vi "Set_valves2.vi"() -> ()   [LabVIEW 2016]
uses:
  ValveGlobals.vi
panel:
  in  "Stop Signal":bool
  out "stop indicator":bool
  in  "Switch Valves":enum16{"1", "2", "3", "4", "5", "6", "7", "8"}[](array[ring])=[enum."6", enum."7"]
  in  "Switch Toggle":bool
  out "Channels 2":bool[][](array[boolean])
  in  "Set Shortcut Pattern":bool
  in  "Clean Cycle Wait Time (s)":u32=8
  in  "Clean Cycle":bool
  in  "Close all Valves":bool
  in  "Set new Values":bool
  in  "stop":bool
  in  "Update Immediately":bool=TRUE
  in  "Which box":string[](array[string])=["A", "B", "C"]
  in  "Channel Nums":string[](array[string])=["1", "2", "3", "4", "5", "6", "7", "8"]
  in  "Channels":bool[][](array[boolean])=[[FALSE, FALSE, FALSE], [FALSE, FALSE, FALSE], [FALSE, FALSE, FALSE], [FALSE, FALSE, FALSE], [FALSE, FALSE, FALSE], [FALSE, FALSE, FALSE], [FALSE, FALSE, FALSE], [FALSE, FALSE, FALSE]]
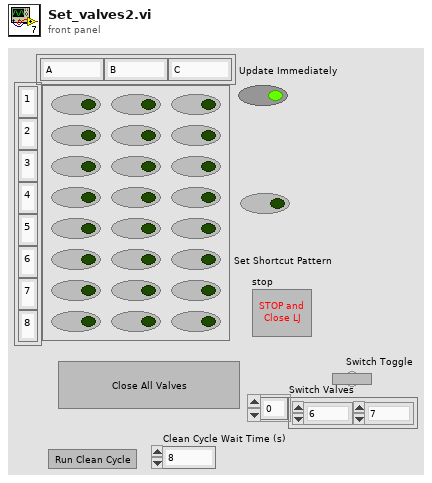
[diagram p1: front panel]
types:
  T1 = enum16{"Release", "Create", "Send", "Wait", "Cancel"}
  T2 = cluster{"Flowboards":enum16{"A", "B", "C"}[], "Channels":enum16{"1", "2", "3", "4", "5", "6", "7", "8"}[], "States":bool[]}
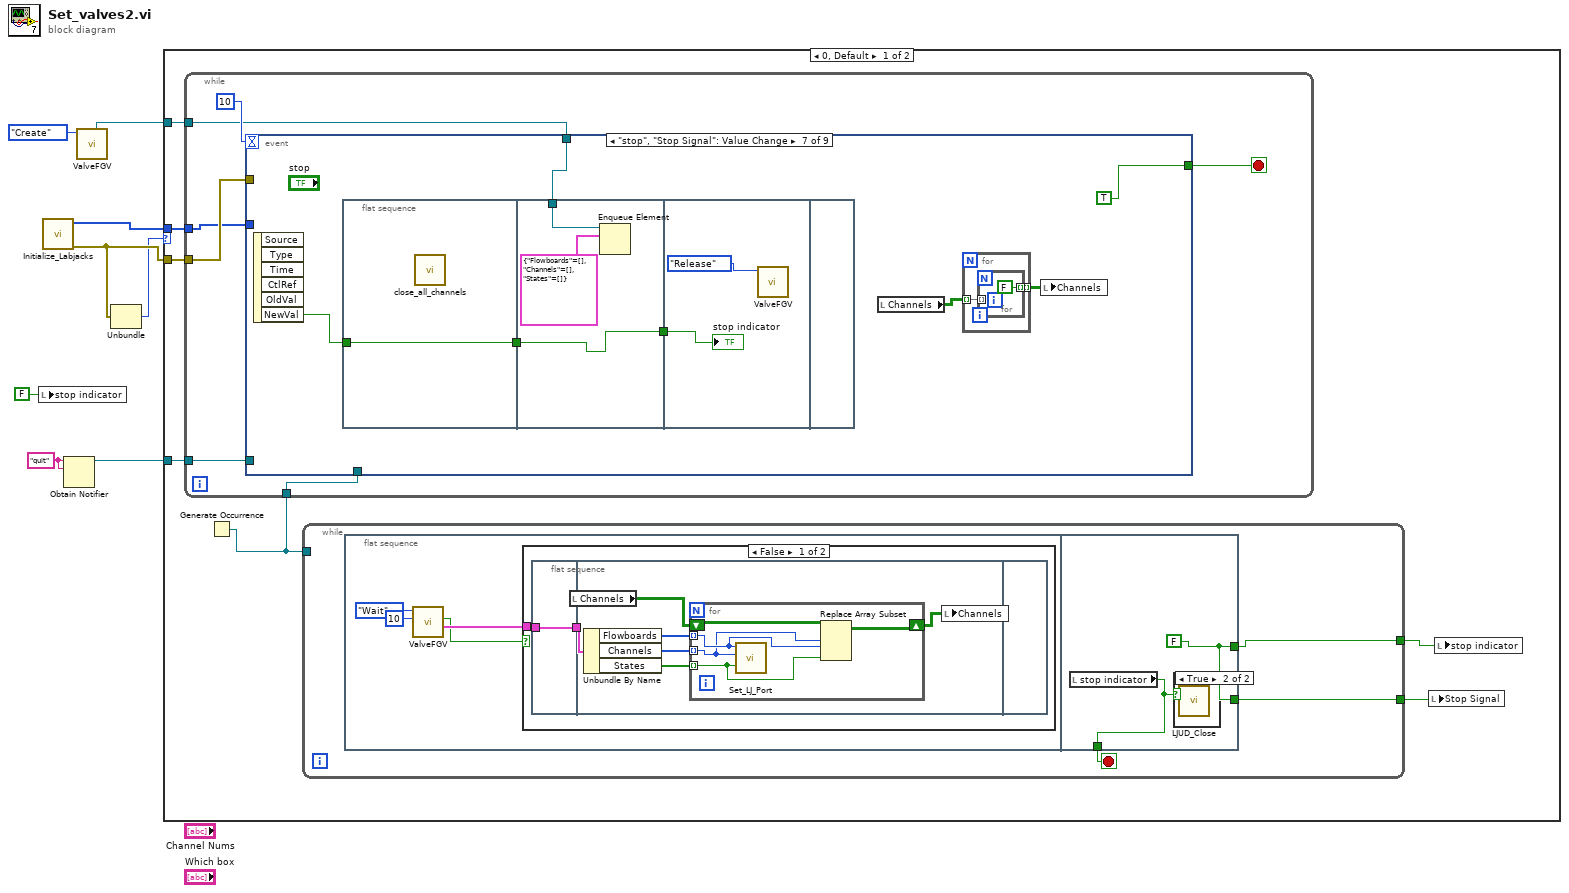
[diagram p0: block diagram]
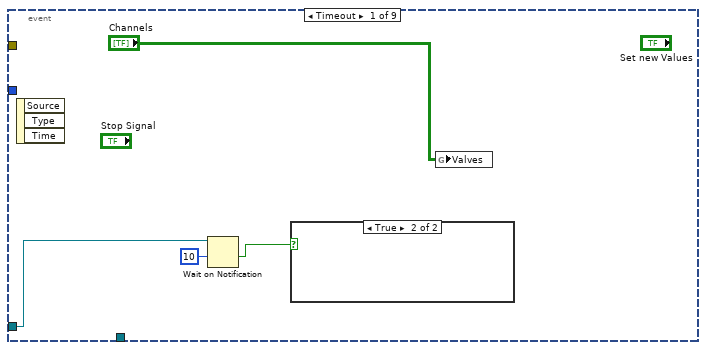
[diagram p4: hidden frame]
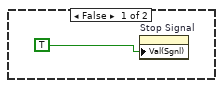
[diagram p5: hidden frame]
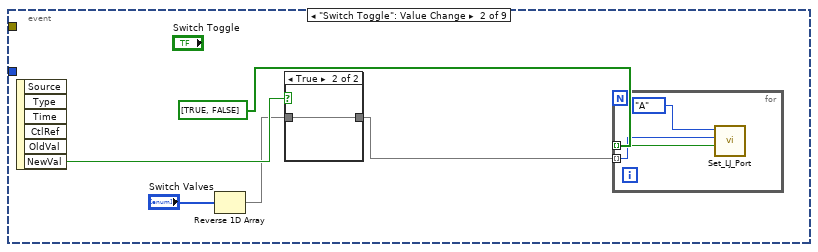
[diagram p6: hidden frame]
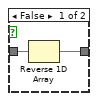
[diagram p7: hidden frame]
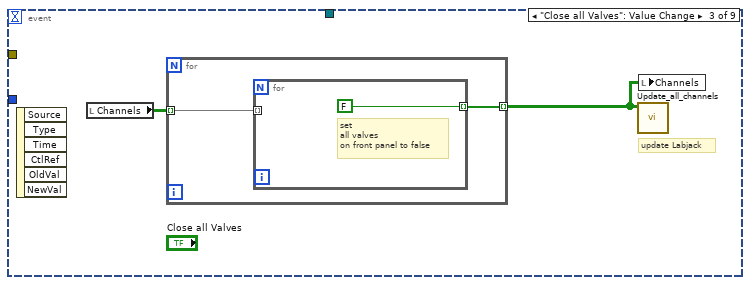
[diagram p8: hidden frame]
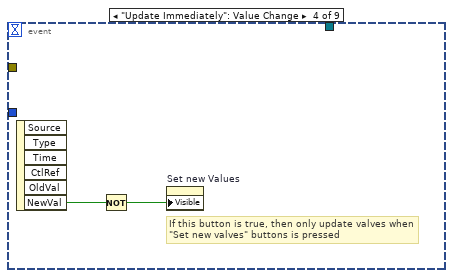
[diagram p9: hidden frame]
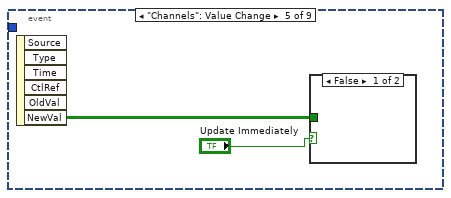
[diagram p10: hidden frame]
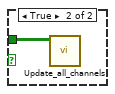
[diagram p11: hidden frame]
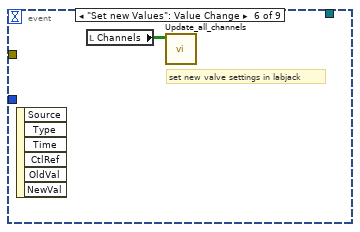
[diagram p12: hidden frame]
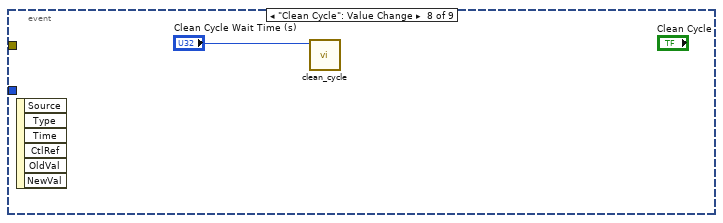
[diagram p13: hidden frame]
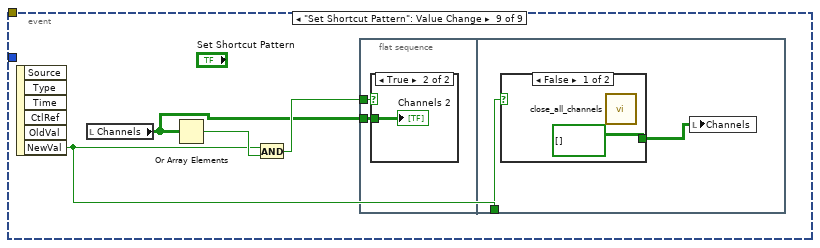
[diagram p14: hidden frame]
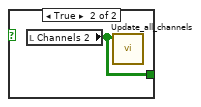
[diagram p16: hidden frame]
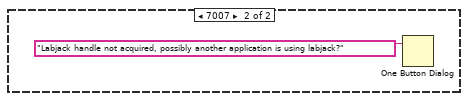
[diagram p17: hidden frame]
diagram:
  w2 = "quit" ("name (unnamed)")
  n1 = local write "stop indicator"(FALSE ("stop indicator")) -> ()
  n2 = call "Initialize_Labjacks.vi"() -> ("error out"=w7:errorcluster, "LJ Handles"=w8:i32[])  [unwired: 10 in]
  n3 = Obtain Notifier(name (unnamed)=w2, notification data type=w2) -> (notifier out=w1:refnum<notifier>)  [unwired: 2 in, 2 out]
  n4 = call "ValveFGV.vi"("Action"=T1."Create") -> ("queue out"=w3:refnum<queue>)  [unwired: 7 in, 3 out]
  n5 = Unbundle(w7) -> ("code"=w6:i32)  [unwired: 2 out]
  n6 = case shown="0, Default" w6 {
    tunnel: w8 -> [w15 _]
    tunnel: w7 -> [w14 _]
    tunnel: w3 -> [w12 _]
    tunnel: w1 -> [w11 _]
    frame 0, Default {
      n7 = Generate Occurrence() -> (w13:refnum<k4>)
      n8 = while {
        tunnel: w15 -> [w43]
        tunnel: w14 -> [w44]
        tunnel: w13 -> [w42]
        tunnel: w12 -> [w41]
        tunnel: w11 -> [w40]
        stop <- w39 stop-if-true
        n9 = event shown="[6] \"stop\", \"Stop Signal\": Value Change" {
          selector: _ -> [_ _ _ _ _ _ _ _ _]
          dyn-events: _ -> [_ _ _ _ _ _ _ _ _]
          timeout: 10 -> [_ _ _ _ _ _ _ _ _]
          tunnel: w44 -> [_ _ _ _ _ _ _ _ _]
          tunnel: w43 -> [_ _ _ _ _ _ _ _ _]
          tunnel: w42 -> [_ _ _ _ _ _ _ _ _]
          tunnel: w41 -> [_ _ _ _ _ _ w78 _ _]
          tunnel: w40 -> [w48 _ _ _ _ _ _ _ _]
          tunnel: [_ _ _ _ _ _ TRUE _ _] -> w39
          event Timeout {
            n10 = event-data() -> ()  [unwired: 1 in, 3 out]
            n11 = Wait on Notification(notifier=w48, timeout in ms (-1)=10) -> (timed out?=w46:bool)  [unwired: 2 in, 3 out]
            n12 = case shown="True" w46 {
              frame False {
                n13 = property on="Stop Signal" class="Bool (strict)"("Val(Sgnl)"=TRUE ("Value (Signaling)")) -> ()  [unwired: 2 in, 2 out]
              }
              frame True {
              }
            }
            n14 = global write "ValveGlobals.vi" "Valves"("Channels") -> ()
          }
          event "Switch Toggle": Value Change {
            n15 = event-data() -> ("NewVal"=w55:bool)  [unwired: 1 in, 5 out]
            n16 = Reverse 1D Array(array="Switch Valves") -> (reversed array=w51:enum16{"1", "2", "3", "4", "5", "6", "7", "8"}[])
            n17 = case shown="True" w55 {
              tunnel: w51 -> [w60 w61]
              tunnel: [w59 w61] -> w53
              frame False {
                n18 = Reverse 1D Array(array=w60) -> (reversed array=w59:enum16{"1", "2", "3", "4", "5", "6", "7", "8"}[])
              }
              frame True {
              }
            }
            n19 = for {
              tunnel: w53 -> [w58] mode=indexing
              tunnel: bool[] [TRUE, FALSE] ("Boards") -> [w56] mode=indexing
              n20 = call "Set_LJ_Port.vi"("State"=w56, "Channel"=w58, "Flowboard"=enum16{"A", "B", "C"}."A") -> ()  [unwired: 8 in, 1 out]
            }
          }
          event "Close all Valves": Value Change {
            # "update Labjack"
            n21 = event-data() -> ()  [unwired: 1 in, 6 out]
            n22 = local read "Channels"() -> (w63:bool[][])
            n23 = for {
              tunnel: w63 -> [w65] mode=indexing
              tunnel: [w64] -> w62 mode=indexing
              n24 = for {
                tunnel: w65 -> [_] mode=indexing
                tunnel: [FALSE] -> w64 mode=indexing
                # "set\nall valves\non front panel to false"
              }
            }
            n25 = call "Update_all_channels.vi"("Channel Values"=w62) -> ()  [unwired: 11 in]
            n26 = local write "Channels"(w62) -> ()
          }
          event "Update Immediately": Value Change {
            # "If this button is true, then only update valves when\n\"Set new valves\" buttons is pressed"
            n27 = event-data() -> ("NewVal"=w68:bool)  [unwired: 1 in, 5 out]
            n28 = Not(x=w68) -> (.not. x?=w67:bool)
            n29 = property on="Set new Values" class="Bool (strict)"("Visible"=w67) -> ()  [unwired: 2 in, 2 out]
          }
          event "Channels": Value Change {
            n30 = event-data() -> ("NewVal"=w69:bool[][])  [unwired: 1 in, 5 out]
            n31 = case shown="False" "Update Immediately" {
              tunnel: w69 -> [_ w71]
              frame False {
              }
              frame True {
                n32 = call "Update_all_channels.vi"("Channel Values"=w71) -> ()  [unwired: 11 in]
              }
            }
          }
          event "Set new Values": Value Change {
            # "set new valve settings in labjack"
            n33 = event-data() -> ()  [unwired: 1 in, 6 out]
            n34 = local read "Channels"() -> (w72:bool[][])
            n35 = call "Update_all_channels.vi"("Channel Values"=w72) -> ()  [unwired: 11 in]
          }
          event "stop", "Stop Signal": Value Change {
            n36 = event-data() -> ("NewVal"=w79:bool)  [unwired: 1 in, 5 out]
            n37 = flat-sequence {
              tunnel: w79 -> [w83]
              tunnel: [w83] -> w74
              tunnel: w78 -> [w86]
              tunnel: w74 -> [w84]
              tunnel: [w84] -> w73
              tunnel: w73 -> [w87]
              frame #0 {
                n38 = call "close_all_channels.vi"() -> ()  [unwired: 12 in]
              }
              frame #1 {
                n39 = Enqueue Element(queue=w86, element=T2 {"Flowboards"=[], "Channels"=[], "States"=[]} ("Valve Data")) -> ()  [unwired: 2 in, 3 out]
              }
              frame #2 {
                n40 = call "ValveFGV.vi"("Action"=T1."Release") -> ()  [unwired: 7 in, 4 out]
                "stop indicator" <- w87
              }
              frame #3 {
              }
            }
            n41 = local read "Channels"() -> (w75:bool[][])
            n42 = for {
              tunnel: [w81] -> w76 mode=indexing
              tunnel: w75 -> [w80] mode=indexing
              n43 = for {
                tunnel: [FALSE] -> w81 mode=indexing
                tunnel: w80 -> [_] mode=indexing
              }
            }
            n44 = local write "Channels"(w76) -> ()
          }
          event "Clean Cycle": Value Change {
            n45 = event-data() -> ()  [unwired: 1 in, 6 out]
            n46 = call "clean_cycle.vi"("seconds to wait"="Clean Cycle Wait Time (s)") -> ()  [unwired: 11 in]
          }
          event "Set Shortcut Pattern": Value Change {
            n47 = event-data() -> ("NewVal"=w90:bool)  [unwired: 1 in, 5 out]
            n48 = local read "Channels"() -> (w91:bool[][])
            n49 = Or Array Elements(Boolean array=w91) -> (logical OR=w93:bool)
            n50 = And(x=w90, y=w93) -> (x .and. y?=w92:bool)
            n51 = flat-sequence {
              tunnel: w92 -> [w95]
              tunnel: w91 -> [w94]
              tunnel: w90 -> [w98]
              frame #0 {
                n52 = case shown="True" w95 {
                  tunnel: w94 -> [_ w96]
                  frame False {
                  }
                  frame True {
                    "Channels 2" <- w96
                  }
                }
              }
              frame #1 {
                n53 = case shown="False" w98 {
                  tunnel: [bool[][] [] ("Channels 2") w100] -> w97
                  frame False {
                    n54 = call "close_all_channels.vi"() -> ()  [unwired: 12 in]
                  }
                  frame True {
                    n55 = local read "Channels 2"() -> (w100:bool[][])
                    n56 = call "Update_all_channels.vi"("Channel Values"=w100) -> ()  [unwired: 11 in]
                  }
                }
                n57 = local write "Channels"(w97) -> ()
              }
            }
          }
        }
      }
      n58 = while {
        tunnel: w13 -> [_]
        tunnel: [w17] -> w10
        tunnel: [w16] -> w9
        stop <- w18 stop-if-true
        n59 = flat-sequence {
          tunnel: [w37] -> w18
          tunnel: [w38] -> w17
          tunnel: [w38] -> w16
          frame #0 {
            n60 = call "ValveFGV.vi"("timeout in ms (-1)"=10, "Action"=T1."Wait") -> ("Valve Data Out"=w22:T2, "timed out?"=w19:bool)  [unwired: 6 in, 2 out]
            n61 = case shown="False" w19 {
              tunnel: w22 -> [w24 _]
              frame False {
                n62 = flat-sequence {
                  tunnel: w24 -> [w25]
                  tunnel: [w25] -> w23
                  tunnel: w23 -> [w26]
                  frame #0 {
                  }
                  frame #1 {
                    n63 = local read "Channels"() -> (w28:bool[][])
                    n64 = Unbundle By Name(w26) -> ("Flowboards"=w31:enum16{"A", "B", "C"}[], "Channels"=w30:enum16{"1", "2", "3", "4", "5", "6", "7", "8"}[], "States"=w29:bool[])
                    n65 = for {
                      tunnel: w31 -> [w35] mode=indexing
                      tunnel: w30 -> [w34] mode=indexing
                      tunnel: w29 -> [w33] mode=indexing
                      shift-right: [w32] -> w27
                      shift-left: w28 -> [w36]
                      n66 = call "Set_LJ_Port.vi"("State"=w33, "Channel"=w34, "Flowboard"=w35) -> ()  [unwired: 8 in, 1 out]
                      n67 = Replace Array Subset(array=w36, new element=w33, index (row)=w34, index (col)=w35) -> (w32:bool[][])
                    }
                    n68 = local write "Channels"(w27) -> ()
                  }
                  frame #2 {
                  }
                }
              }
              frame True {
              }
            }
          }
          frame #1 {
            w38 = FALSE ("stop indicator")
            n69 = local read "stop indicator"() -> (w37:bool)
            n70 = case shown="True" w37 {
              frame False {
              }
              frame True {
                n71 = call "LJUD_Close.vi"() -> ()  [unwired: 11 in, 1 out]
              }
            }
          }
        }
      }
      n72 = local write "Stop Signal"(w9) -> ()
      n73 = local write "stop indicator"(w10) -> ()
    }
    frame 7007 {
      n74 = One Button Dialog(message="Labjack handle not acquired, possibly another application is using labjack?") -> ()  [unwired: 1 in, 1 out]
    }
  }
